vi "FindMaxZ.vi"(11 "cmd amd State":cluster{"Command":string, "End State":dbl[]}[](array[cluster])) -> (1 "Z Colors":u32[](array[numeric]), 2 "Array":dbl[](array[numeric]), 3 "Max":dbl, 5 "Cutting Bounds":T1 {"Z Max" format="%#.1f"; "Z Min" format="%#.1f"; "Y Max" format="%#.1f"; "Y Min" format="%#.1f"; "X Max" format="%#.1f"; "X Min" format="%#.1f"})   [LabVIEW 2023]
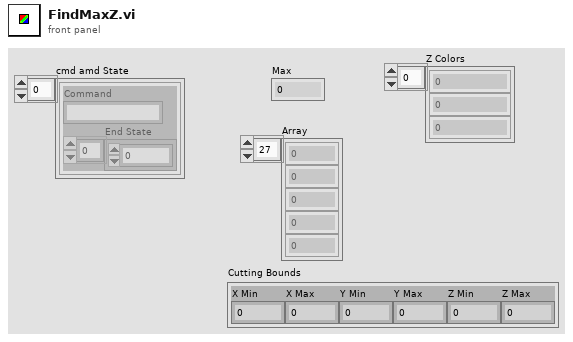
[diagram p1: front panel]
types:
  T1 = cluster{"X Min":dbl, "X Max":dbl, "Y Min":dbl, "Y Max":dbl, "Z Min":dbl, "Z Max":dbl}
  T2 = enum16{"Apricot", "Carnation", "Ether", "Greyscale", "Greyscale-banded", "Hot Metal", "Lava Waves", "Mac", "Morning Glory", "Rainbow", "Rainbow-banded", "Rainbow-inverted", "Rainbow-striped", "Saturn", "Seismic", "Space"}
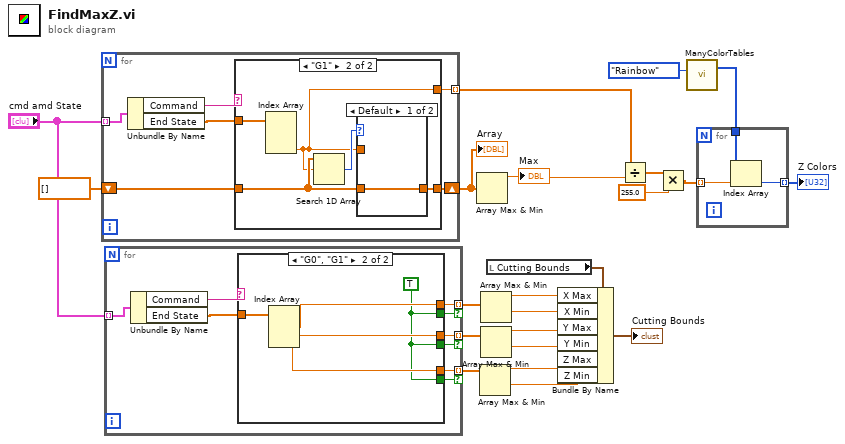
[diagram p0: block diagram]
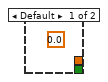
[diagram p2: hidden frame]
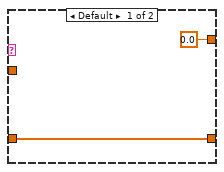
[diagram p3: hidden frame]
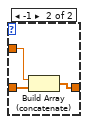
[diagram p4: hidden frame]
diagram:
  n1 = for {
    tunnel: "cmd amd State" -> [w28] mode=indexing
    shift-right: [w26] -> w22
    shift-left: dbl[] [] -> [w25]
    tunnel: [w24] -> w18 mode=indexing
    n2 = Unbundle By Name(w28) -> ("Command"=w23:string, "End State"=w27:dbl[])
    n3 = case shown="\"G1\"" w23 {
      tunnel: w27 -> [_ w35]
      tunnel: [w30 w33] -> w26
      tunnel: w25 -> [w30 w32]
      tunnel: [0.0 w31] -> w24
      frame Default {
      }
      frame "G1" {
        n4 = Index Array(array=w35) -> (element #3=w31:dbl)  [unwired: 3 in, 2 out]
        n5 = Search 1D Array(1D array=w32, element=w31) -> (index of element=w34:i32)  [unwired: 1 in]
        n6 = case shown="Default" w34 {
          tunnel: [w36 w37] -> w33
          tunnel: w32 -> [w36 w39]
          tunnel: w31 -> [_ w38]
          frame Default {
          }
          frame -1 {
            n7 = Build Array (concatenate)(w38, w39) -> (w37:dbl[])
          }
        }
      }
    }
  }
  "Array" <- w22
  n8 = for {
    tunnel: "cmd amd State" -> [w48] mode=indexing
    tunnel: [w45] -> w11 mode=indexing if=w42
    tunnel: [w44] -> w10 mode=indexing if=w41
    tunnel: [w43] -> w9 mode=indexing if=w40
    n9 = Unbundle By Name(w48) -> ("Command"=w46:string, "End State"=w47:dbl[])
    n10 = case shown="\"G0\", \"G1\"" w46 {
      tunnel: w47 -> [_ w53]
      tunnel: [_ w52] -> w45
      tunnel: [_ w51] -> w44
      tunnel: [_ w50] -> w43
      tunnel: [_ w49] -> w42
      tunnel: [_ w49] -> w41
      tunnel: [_ w49] -> w40
      frame Default {
        (unwired) 0.0
      }
      frame "G0", "G1" {
        w49 = TRUE
        n11 = Index Array(array=w53) -> (element #1=w52:dbl, element #2=w51:dbl, element #3=w50:dbl)  [unwired: 3 in]
      }
    }
  }
  n12 = Array Max & Min(array=w22) -> (max value=w17:dbl)  [unwired: 3 out]
  "Max" <- w17
  n13 = Array Max & Min(array=w9) -> (max value=w6:dbl, min value=w7:dbl)  [unwired: 2 out]
  n14 = Array Max & Min(array=w11) -> (max value=w2:dbl, min value=w3:dbl)  [unwired: 2 out]
  n15 = Array Max & Min(array=w10) -> (max value=w4:dbl, min value=w5:dbl)  [unwired: 2 out]
  n16 = local read "Cutting Bounds"() -> (w8:T1)
  n17 = Bundle By Name(cluster=w8, "X Max"=w2, "X Min"=w3, "Y Max"=w4, "Y Min"=w5, "Z Max"=w6, "Z Min"=w7) -> (→"Cutting Bounds":T1)
  n18 = Divide(x=w18, y=w17) -> (x/y=w20:dbl[])
  n19 = Multiply(x=w20, y=255.0) -> (x*y=w14:dbl[])
  n20 = call "ManyColorTables.vi"("Color Table"=T2."Rainbow") -> ("Color Table Out"=w15:u32[])  [unwired: 2 in]
  n21 = for {
    tunnel: w15 -> [w56]
    tunnel: w14 -> [w55] mode=indexing
    tunnel: [w54] -> w13 mode=indexing
    n22 = Index Array(array=w56, index=w55) -> (element=w54:u32)
  }
  "Z Colors" <- w13
